vi "DelFrmXYGrphCrvsBatch.vi"(8 "error in (no error)":errorcluster caption="entrée d'erreur (pas d'erreur)", 9 "CurvIndex":i32[](array[numeric]), 10 "GraphIndex":i32[](array[numeric]), 11 "Interface en entrée":refnum<class "Interface.lvclass"> caption="DNL_LabVIEW Object in") -> (0 "error out":errorcluster caption="sortie d'erreur", 3 "Interface en sortie":refnum<class "Interface.lvclass"> caption="DNL_LabVIEW Object out")   [LabVIEW 2019, in "Interface.lvclass"]
uses:
  Interface.lvclass
  Interface.lvclass/Interface.ctl
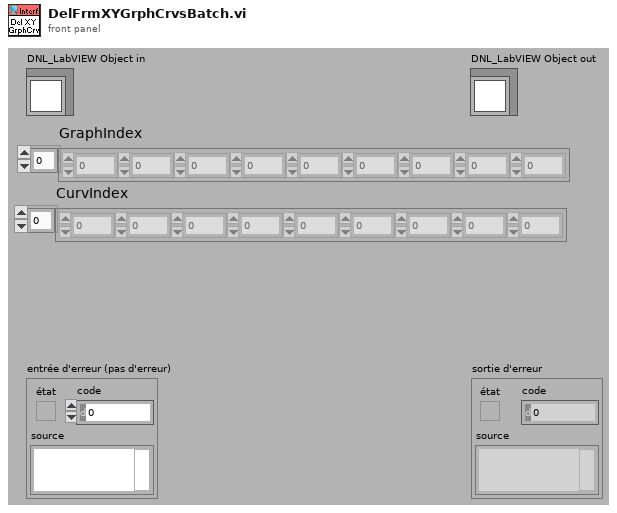
[diagram p1: front panel]
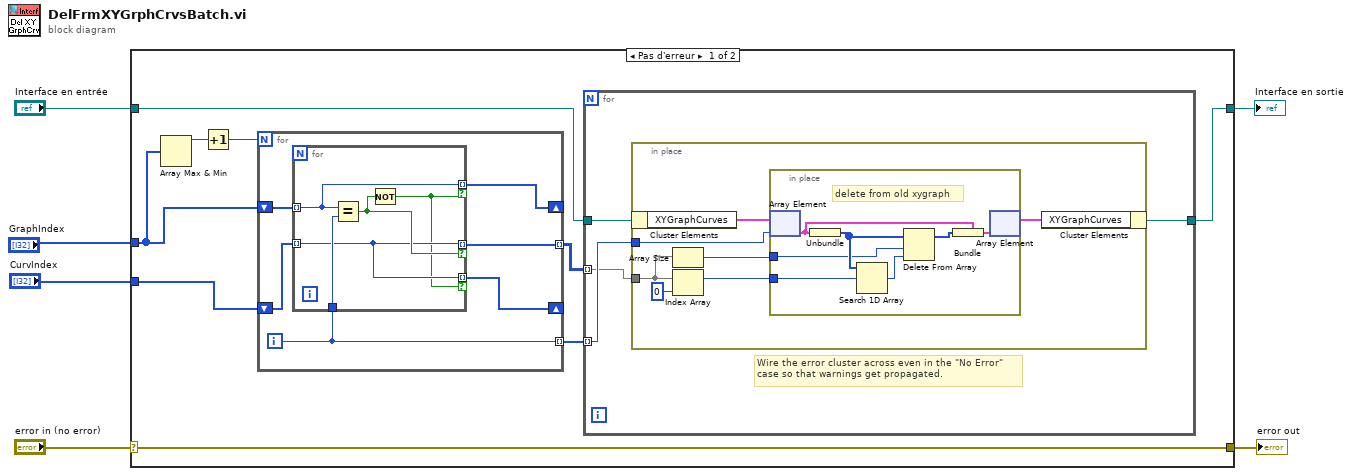
[diagram p0: block diagram]
diagram:
  n1 = case shown="Pas d'erreur" "error in (no error)" {
    selector: "error in (no error)" -> [w15 w46]
    tunnel: [w15 w46] -> w5
    tunnel: [w13 w45] -> w3
    tunnel: "Interface en entrée" -> [w14 w45]
    tunnel: "CurvIndex" -> [w11 _]
    tunnel: "GraphIndex" -> [w12 _]
    frame No Error {
      n2 = Array Max & Min(array=w12) -> (max value=w10:i32)  [unwired: 3 out]
      n3 = Increment(x=w10) -> (x+1=w7:i32)
      n4 = for {
        N: w7 -> [_]
        tunnel: [w39] -> w8 mode=indexing
        shift-right: [w35] -> _
        shift-left: w11 -> [w37]
        shift-right: [w36] -> _
        shift-left: w12 -> [w38]
        tunnel: [w34] -> w9 mode=indexing
        i -> [w34]
        n5 = for {
          tunnel: w38 -> [w42] mode=indexing
          tunnel: w34 -> [w44]
          tunnel: w37 -> [w41] mode=indexing
          tunnel: [w41] -> w39 mode=indexing if=w43
          tunnel: [w42] -> w36 mode=indexing if=w40
          tunnel: [w41] -> w35 mode=indexing if=w40
          n6 = Equal?(x=w42, y=w44) -> (x = y?=w43:bool)
          n7 = Not(x=w43) -> (.not. x?=w40:bool)
        }
      }
      n8 = for {
        tunnel: w14 -> [w19]
        tunnel: [w18] -> w13
        tunnel: w9 -> [w17] mode=indexing
        tunnel: w8 -> [w16] mode=indexing
        # "Wire the error cluster across even in the \"No Error\"\ncase so that warnings get propagated."
        n9 = in-place {
          in-place-border: w16 -> [w21]
          in-place-border: w17 -> [w25]
          n10 = in-place-cluster #1(w19) -> ("XYGraphCurves"=w26:cluster{"Tableau":i32[]}[])
          n11 = Array Size(array=w21) -> (size(s)=w20:i32)
          n12 = Index Array(array=w21, index=0 ("indice")) -> (element=w23:i32)
          n13 = in-place {
            in-place-border: w23 -> [w28]
            in-place-border: w20 -> [w27]
            # "delete from old xygraph"
            n14 = in-place-array #2(w26, w25) -> (w31:cluster{"Tableau":i32[]})
            n15 = Unbundle(w31) -> ("Tableau"=w32:i32[])
            n16 = Search 1D Array(1D array=w32, element=w28) -> (index of element=w33:i32)  [unwired: 1 in]
            n17 = Delete From Array(array=w32, length=w27, index=w33) -> (array with subset deleted=w29:i32[])  [unwired: 1 out]
            n18 = Bundle(cluster=w31, "Tableau"=w29) -> (w30:cluster{"Tableau":i32[]})
            n19 = in-place-array #2(w30) -> (w24:cluster{"Tableau":i32[]}[])  [unwired: 1 out]
          }
          n20 = in-place-cluster #1("XYGraphCurves"=w24) -> (w18:refnum<class "Interface.lvclass">)
        }
      }
    }
    frame Error {
    }
  }
  "error out" <- w5
  "Interface en sortie" <- w3
